vi "H5Glink2.vi"(6 "Link Type":T2 items=["H5G_LINK_ERROR"=-1, "H5G_LINK_HARD"=0, "H5G_LINK_SOFT"=1], 7 "HDF5 New Loc (same)":T1, 8 "error in (no error)":errorcluster, 9 "New Name":string, 10 "Current Name":string, 11 "HDF5 Ref":T1) -> (0 "error out":errorcluster, 3 "HDF5 Ref out":T1)   [LabVIEW 2017]
doc: "This function is deprecated in favor of the functions \n H5Lcreate_hard\n and\n H5Lcreate_soft."
uses:
  <vilib>/UPVI/lvhdf5/library.llb/HDF5 Ref.ctl
  <vilib>/UPVI/lvhdf5/group.llb/H5G_link_t.ctl
  <vilib>/UPVI/lvhdf5/hdf5.dll
panel:
  # "LVHDF5 Toolkit\nCopyright (c) 2005-2013 by Jason D. Sommerville\nCopyright (c) 2014 by UPVI, LLC.\n\nThis use and distribution of this file is governed by the terms found in \nLICENSE.txt distributed with this toolkit and installed at\n <user.lib>\\_lvhdf5\\LICENSE.txt"
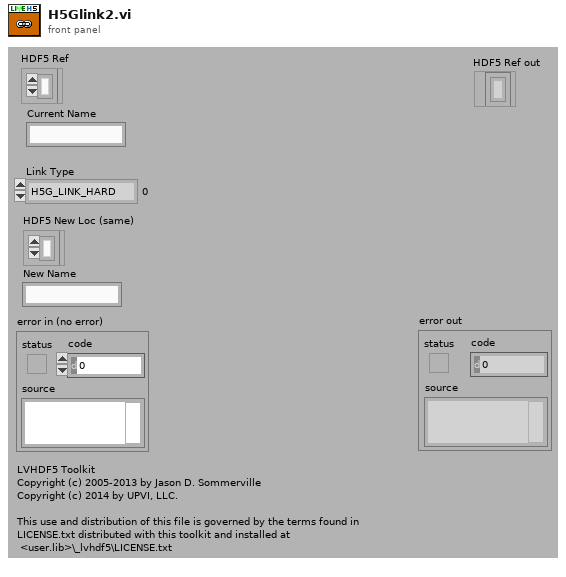
[diagram p1: front panel]
types:
  T1 = typedef "HDF5 Ref.ctl" = refnum<k1>
  T2 = typedef "H5G_link_t.ctl" = i32
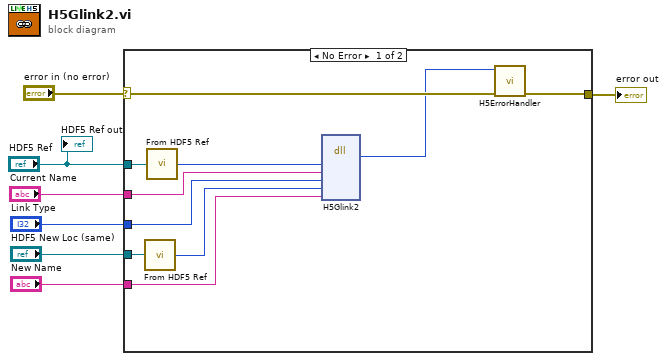
[diagram p0: block diagram]
diagram:
  n1 = case shown="No Error" "error in (no error)" {
    selector: "error in (no error)" -> [w17 w18]
    tunnel: [w16 w18] -> w6
    tunnel: "HDF5 Ref" -> [w14 _]
    tunnel: "Link Type" -> [w10 _]
    tunnel: "Current Name" -> [w11 _]
    tunnel: "New Name" -> [w8 _]
    tunnel: "HDF5 New Loc (same)" -> [w12 _]
    frame No Error {
      n2 = call <vilib>:"From HDF5 Ref.vi"("HDF5 Ref"=w12) -> ("I32"=w9:i32)
      n3 = call <vilib>:"From HDF5 Ref.vi"("HDF5 Ref"=w14) -> ("I32"=w13:i32)
      n4 = dll-call lib="C:/Program Files/National Instruments/LabVIEW 2017/vi.lib/UPVI/lvhdf5/hdf5.dll" fn="H5Glink2"("loc_id"=w13, "current_name"=w11, "link_type"=w10, "new_loc_id"=w9, "new_name"=w8) -> (w15:i32)  [unwired: 8 in, 2 out]
      n5 = call <vilib>:"H5ErrorHandler.vi"("error in (no error)"=w17, "herr_t"=w15) -> ("error out"=w16:errorcluster)  [unwired: 3 in, 4 out]
    }
    frame Error {
    }
  }
  "error out" <- w6
  "HDF5 Ref out" <- "HDF5 Ref"
